vi "Find 0 Crossings.vi"(8 "Error In":errorcluster, 10 "dX/dt":dbl[](array[numeric]), 11 "Intensities":dbl[](array[numeric])=[55.0, 56.0, 46.0, 32.0, 21.0, 37.0, 92.0, 179.0, 213.0, 312.0, 312.0, 297.0, 296.0, 224.0, 192.0, 50.0, 58.0, 96.0, 112.0, 108.0, 107.0, 117.0, 101.0, 79.0, 28.0, 242.0, 3002.0, 4321.0, 6382.0, 8039.0, 8112.0, 7467.0, 6673.0, 6730.0, 4821.0, 161.0, 116.0, 199.0, 280.0, 324.0, 385.0, 306.0, 340.0, 270.0, 209.0, 596.0, 8839.0, 15018.0, 22096.0, 27306.0, 28282.0, 26382.0, 24772.0, 19971.0, 16031.0, 677.0, 291.0, 595.0, 848.0, 1124.0, 1192.0, 1040.0, 1069.0, 767.0, 821.0, 50.0, 66.0, 105.0, 160.0, 163.0, 147.0, 163.0, 127.0, 96.0, 73.0, 9.0, 4.0, 4.0, 19.0, 10.0, 14.0, 8.0, 14.0, 7.0, 9.0, 44.0, 57.0, 86.0, 126.0, 111.0, 98.0, 79.0, 95.0, 67.0, 16.0, 19.0, 17.0, 25.0, 30.0, 39.0, 38.0, 191.0, 275.0, 254.0, 270.0, 293.0, 216.0, 219.0, 170.0, 180.0, 186.0, 212.0, 255.0, 355.0, 365.0, 354.0, 352.0, 389.0, 310.0, 272.0, 208.0, 189.0, 175.0, 203.0, 226.0, 202.0, 206.0, 278.0, 279.0, 414.0, 799.0, 1517.0, 2446.0, 3938.0, 4796.0, 5265.0, 5583.0, 5257.0, 4438.0, 3543.0, 2831.0, 1347.0, 1119.0, 1370.0, 1782.0, 1807.0, 1828.0, 2082.0, 2011.0, 2473.0, 4735.0, 8059.0, 13114.0, 21491.0, 25990.0, 28670.0, 29595.0, 29953.0, 26733.0, 21472.0, 14896.0, 7745.0, 6381.0, 7465.0, 9646.0, 10328.0, 10403.0, 10136.0, 9622.0, 7344.0, 5462.0, 2287.0, 1703.0, 2115.0, 2635.0, 3263.0, 4044.0, 5060.0, 5508.0, 6042.0, 6139.0, 6124.0, 6909.0, 7394.0, 6919.0, 6393.0, 5036.0, 5125.0, 4926.0, 3939.0, 3280.0, 2071.0, 2019.0, 1927.0, 1569.0, 1324.0, 992.0, 958.0, 880.0, 889.0, 993.0, 1241.0, 163.0, 122.0, 143.0, 189.0, 188.0, 214.0, 226.0, 254.0, 230.0, 216.0, 170.0, 164.0, 205.0, 153.0, 204.0, 137.0, 171.0, 163.0, 229.0, 313.0, 468.0, 667.0, 1041.0, 1532.0, 1899.0, 2343.0, 2797.0, 2956.0, 2591.0, 1993.0, 1475.0, 787.0, 702.0, 842.0, 1073.0, 1341.0, 1708.0, 1886.0, 2506.0, 3796.0, 5659.0, 7754.0, 13596.0, 19036.0, 25687.0, 30761.0, 35888.0, 37967.0, 35251.0, 27029.0, 21428.0, 11593.0, 9040.0, 11127.0, 13005.0, 16089.0, 18097.0, 19329.0, 19088.0, 14510.0, 10053.0, 6086.0, 4080.0, 4322.0, 4947.0, 5697.0, 6188.0, 6839.0, 6325.0, 5298.0, 3850.0, 2157.0, 1592.0, 1569.0, 1697.0, 1935.0, 1994.0, 2079.0, 2043.0, 1563.0, 1245.0, 826.0, 516.0, 585.0, 620.0, 609.0, 625.0, 651.0, 677.0, 707.0, 761.0, 879.0, 1091.0, 1597.0, 1813.0, 2074.0, 2314.0, 2176.0, 2032.0, 1570.0, 1155.0, 21.0, 18.0, 5.0, 22.0, 10.0, 11.0, 23.0, 8.0, 11.0, 20.0, 14.0, 12.0, 22.0, 8.0, 12.0, 19.0, 14.0, 16.0, 9.0, 18.0, 12.0, 21.0, 16.0, 22.0, 13.0, 20.0, 13.0, 26.0, 26.0, 44.0, 30.0, 56.0, 52.0, 39.0, 33.0, 26.0, 18.0, 29.0, 34.0, 36.0, 39.0, 47.0, 55.0, 113.0, 124.0, 202.0, 279.0, 355.0, 573.0, 856.0, 1150.0, 1298.0, 1700.0, 1791.0, 1294.0, 1052.0, 874.0, 526.0, 667.0, 865.0, 992.0, 1286.0, 1427.0, 1381.0, 1239.0, 962.0, 662.0, 386.0, 392.0, 452.0, 513.0, 627.0, 706.0, 779.0, 523.0, 425.0, 309.0, 188.0, 172.0, 182.0, 179.0, 207.0, 285.0, 246.0, 231.0, 183.0, 112.0, 65.0, 58.0, 81.0, 73.0, 95.0, 110.0, 112.0, 67.0, 78.0, 79.0, 70.0, 78.0, 92.0, 108.0, 43.0, 40.0, 52.0, 32.0, 53.0, 51.0, 37.0, 35.0, 43.0, 33.0, 39.0, 48.0, 62.0, 38.0, 40.0, 31.0, 42.0, 31.0, 47.0, 41.0, 41.0, 46.0, 49.0, 59.0, 49.0, 56.0, 66.0, 49.0, 57.0, 78.0, 107.0, 139.0, 196.0, 263.0, 350.0, 506.0, 639.0, 850.0, 963.0, 1256.0, 1355.0, 1989.0, 2163.0, 2256.0, 2168.0, 2097.0, 1936.0, 1771.0, 1572.0, 1549.0, 1669.0, 1962.0, 1928.0, 2150.0, 2282.0, 1774.0, 1693.0, 1455.0, 1325.0, 1034.0, 984.0, 993.0, 1120.0, 1284.0, 1002.0, 1042.0, 931.0, 781.0, 614.0, 482.0, 424.0, 448.0, 432.0, 435.0, 521.0, 427.0, 389.0, 344.0, 261.0, 187.0, 173.0, 188.0, 218.0, 209.0, 195.0, 185.0, 181.0, 196.0, 212.0, 193.0, 240.0, 203.0, 266.0, 287.0, 280.0, 229.0, 230.0, 207.0, 196.0, 189.0, 180.0, 4.0, 10.0, 7.0, 13.0, 5.0, 15.0, 7.0, 3.0, 13.0, 8.0, 7.0, 8.0, 4.0, 12.0, 11.0, 4.0, 4.0, 11.0, 4.0, 6.0, 8.0, 1.0, 9.0, 11.0, 9.0, 7.0, 8.0, 16.0, 10.0, 13.0, 4.0, 6.0, 10.0, 10.0, 11.0, 15.0, 7.0, 9.0, 6.0, 7.0, 8.0, 16.0, 6.0, 12.0, 7.0, 16.0, 22.0, 63.0, 99.0, 111.0, 172.0, 250.0, 327.0, 379.0, 389.0, 354.0, 296.0, 269.0, 251.0, 177.0, 211.0, 221.0, 341.0, 372.0, 363.0, 332.0, 304.0, 314.0, 240.0, 145.0, 137.0, 169.0, 201.0, 238.0, 259.0, 183.0, 200.0, 192.0, 92.0, 77.0, 60.0, 91.0, 68.0, 87.0, 129.0, 90.0, 88.0, 76.0, 59.0, 28.0, 26.0, 22.0, 36.0, 33.0, 36.0, 47.0, 33.0, 41.0, 31.0, 38.0, 29.0]) -> (0 "Error Out":errorcluster, 3 "Peaks Info":T1[](array[typedef]))   [LabVIEW 2015]
uses:
  Server/AutoCal/Controls/PeakInfoPresenter.ctl
  <vilib>/ptbypt/NI_PtbyPt.lvlib
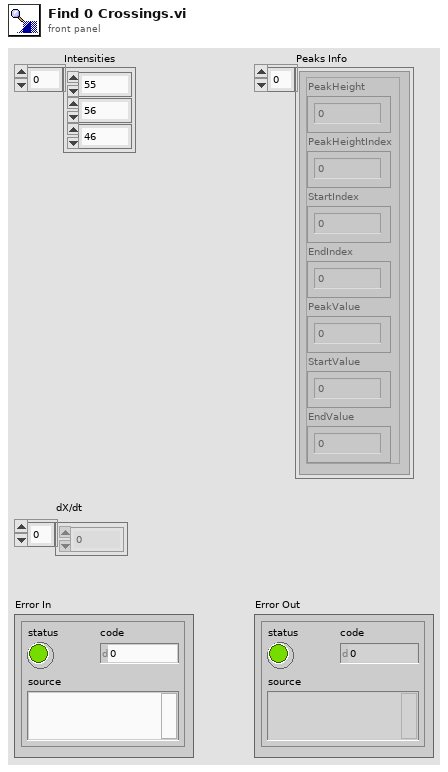
[diagram p1: front panel]
types:
  T1 = typedef "PeakInfoPresenter.ctl" = cluster{"PeakHeight":dbl, "PeakHeightIndex":dbl, "StartIndex":dbl, "EndIndex":dbl, "PeakValue":dbl, "StartValue":dbl, "EndValue":dbl}
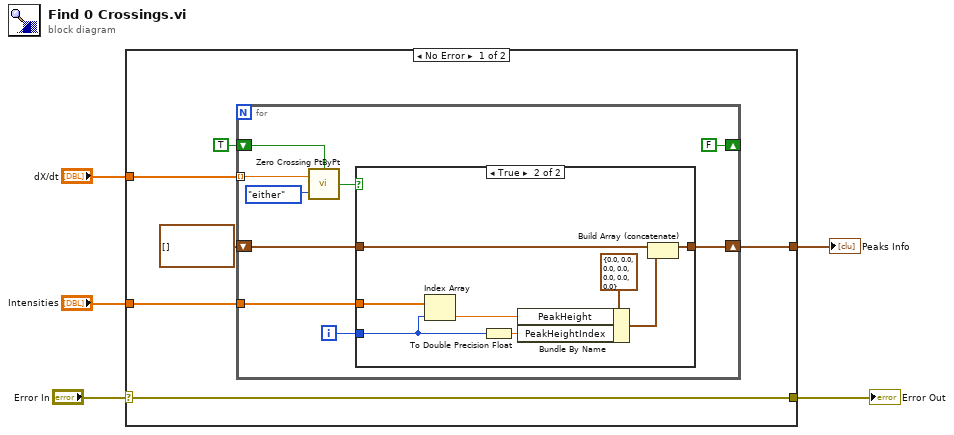
[diagram p0: block diagram]
diagram:
  n1 = case shown="No Error" "Error In" {
    selector: "Error In" -> [w6 w30]
    tunnel: "dX/dt" -> [w11 _]
    tunnel: [w9 _] -> w4
    tunnel: "Intensities" -> [w7 _]
    tunnel: [w6 w30] -> w1
    frame No Error {
      n2 = for {
        tunnel: w11 -> [w20] mode=indexing
        shift-right: [w17] -> w9
        shift-left: T1[] [] ("Array") -> [w18]
        shift-right: [FALSE ("initialize")] -> _
        shift-left: TRUE ("initialize") -> [w14]
        tunnel: w7 -> [w12]
        i -> [w16]
        n3 = call <vilib>:"Zero Crossing PtByPt.vi"("initialize"=w14, "direction"=enum16{"either", "minus-plus", "plus-minus"}."either", "input data point"=w20) -> ("crossing"=w19:bool)
        n4 = case shown="True" w19 {
          tunnel: w18 -> [w21 w28]
          tunnel: [w21 w27] -> w17
          tunnel: w16 -> [_ w22]
          tunnel: w12 -> [_ w25]
          frame False {
          }
          frame True {
            n5 = Index Array(array=w25, index=w22) -> (element=w24:dbl)
            n6 = To Double Precision Float(number=w22) -> (double precision float=w23:dbl)
            n7 = Bundle By Name(cluster=T1 {"PeakHeight"=0.0, "PeakHeightIndex"=0.0, "StartIndex"=0.0, "EndIndex"=0.0, "PeakValue"=0.0, "StartValue"=0.0, "EndValue"=0.0} ("Cluster"), "PeakHeight"=w24, "PeakHeightIndex"=w23) -> (w26:T1)
            n8 = Build Array (concatenate)(w28, w26) -> (w27:T1[])
          }
        }
      }
    }
    frame Error {
    }
  }
  "Peaks Info" <- w4
  "Error Out" <- w1
